vi "Update.vi"(8 "error in (no error)":errorcluster, 10 "Panel Data":variant, 11 "Window Updater in":refnum<class "Window Updater.lvclass">) -> (0 "error out":errorcluster)   [LabVIEW 2020, in "Panel.lvlib" / "Window Updater.lvclass"]
doc: "Updates the Panel from the Panel Data. This will set the VI's Title to the value of the \"Title\" field.\n----\nCopyright: MGI 2017\nAuthor: Derek Trepanier"
uses:
  <vilib>/MGI/Panel Manager/Panel/Panel Updater/Window Updater/Window Updater.lvclass
  <vilib>/MGI/Panel Manager/Panel/Panel Updater/Window Updater/Window Updater.lvclass/Window Updater.ctl
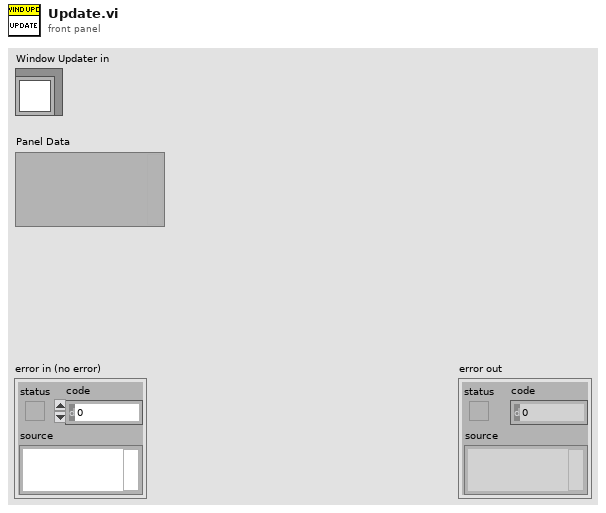
[diagram p1: front panel]
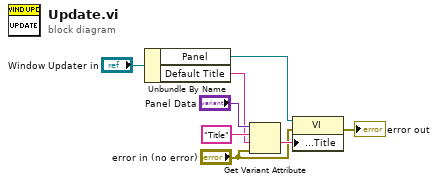
[diagram p0: block diagram]
diagram:
  n1 = Unbundle By Name("Window Updater in") -> ("Panel"=w6:refnum<vi>, "Default Title"=w4:string)
  n2 = Get Variant Attribute(Variant="Panel Data", name="Title", default value (empty Variant)=w4, error in="error in (no error)") -> (value=w3:string)  [unwired: 3 out]
  n3 = property class="VI"(reference=w6, error in="error in (no error)", "Front Panel.Title"=w3) -> (error out=→"error out":errorcluster)  [unwired: 1 out]
